vi "MeasureRMSJ&J.vi"(9 "#of Samples":dbl, 10 "Sampling Rate":dbl) -> (1 "(Vrms)":dbl format="%0.2f", 2 "Waveform Graph":dynamicdata(graph))   [LabVIEW 2015]
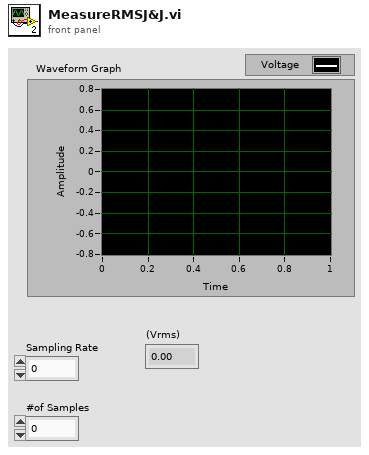
[diagram p1: front panel]
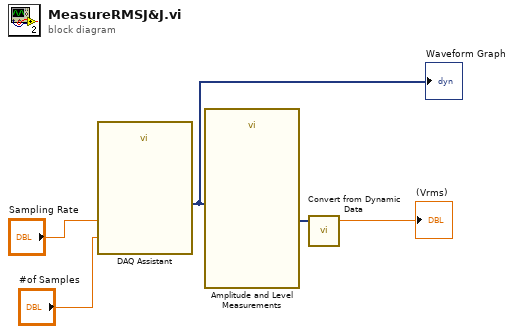
[diagram p0: block diagram]
diagram:
  n1 = call "DAQ Assistant"("rate"="Sampling Rate", "number of samples"="#of Samples") -> ("data"=w1:dynamicdata)  [unwired: 15 in, 2 out]
  "Waveform Graph" <- w1
  n2 = call "Amplitude and Level Measurements"("Signals"=w1) -> ("RMS"=w3:dynamicdata)  [unwired: 13 in, 1 out]
  n3 = call "Convert from Dynamic Data"("Dynamic Data Type"=w3) -> ("Scalar"=→"(Vrms)":dbl)  [unwired: 3 in]
